vi "Help Message Top--constant.vi"() -> (3 "Help Message Top":string)   [LabVIEW 2025]
doc: "This constant contains the initial part of the help message."
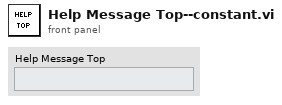
[diagram p1: front panel]
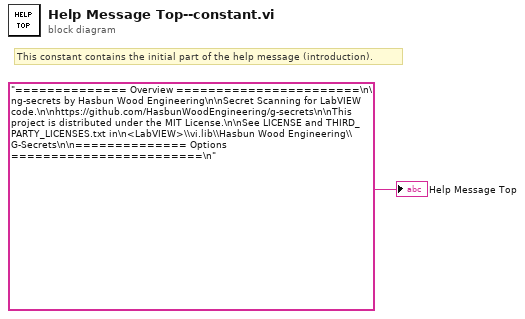
[diagram p0: block diagram]
diagram:
  # "This constant contains the initial part of the help message (introduction)."
  "Help Message Top" <- "============== Overview =======================\n\ng-secrets by Hasbun Wood Engineering\n\nSecret Scanning for LabVIEW code.\n\nhttps://github.com/HasbunWoodEngineering/g-secrets\n\nThis project is distributed under the MIT License.\n\nSee LICENSE and THIRD_PARTY_LICENSES.txt in\n<LabVIEW>\\vi.lib\\Hasbun Wood Engineering\\G-Secrets\n\n============== Options ========================\n"
